vi "MC.SetWavelength.vi"(8 "error in (no error)":errorcluster, 10 "Wavelength, nm":T1, 11 "Measurement.Free":refnum<class "Measurement.Free.lvclass">) -> (0 "error out":errorcluster, 3 "Measurement.Free out":refnum<class "Measurement.Free.lvclass">)   [LabVIEW 2017, in "Measurement.Free.lvclass"]
doc: "---------------------------------------------------------------\nJKI State Machine Objects™\nhttp://jki.net/state-machine-objects/\nCopyright (C) 2005-2015, JKI <info@jki.net>\nALL RIGHTS RESERVEDJKI State Machine Objects (SMO) 1.0.0.4\nJKI - JKI\nCopyright (c) 2015, JKI"
uses:
  Measurement.Free.lvclass
  Typedefs/PrivateEvents--Measurement.Free.MC.SetWavelength.ctl
  Measurement.Free.lvclass/Measurement.Free.ctl
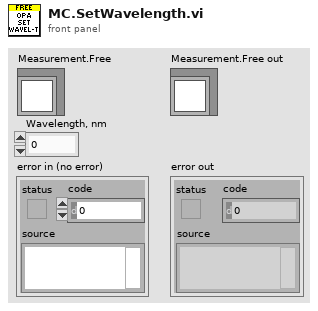
[diagram p1: front panel]
types:
  T1 = typedef "Measurement.Free.lvclass/PrivateEvents--Measurement.Free.MC.SetWavelength.ctl" = dbl
  T2 = typedef "Measurement.Free.lvclass/PrivateData--Ref.ctl" = refnum<data-value>
  T3 = typedef "Measurement.Free.lvclass/PrivateData--Cluster.ctl" = cluster{"Configuration":T4, "Dependencies":T17, "Private Events":T18}
  T4 = typedef "Measurement.Free.lvclass/Configuration--Cluster.ctl" = cluster{"Measurement.Type":T5, "Hardware":T6}
  T5 = typedef "Measurement.lvclass/Measurement.Type--Enum.ctl" = enum16{"Free", "I/V Curve", "Wavelength sweeping", "Photocurrent mapping"}
  T6 = typedef "Measurement.Free.lvclass/Configuration.Hardware--Cluster.ctl" = cluster{"SMU":T7, "LIA":T9, "OPM":T11, "OPA":T13, "MC":T15}
  T7 = typedef "Measurement.lvclass/Configuration.SMU--Cluster.ctl" = cluster{"Enable":bool, "SMU Model":string, "Configuration":T8}
  T8 = typedef "SMU.lvclass/Configuration--Cluster.ctl" = cluster{"VISA Resource":string, "Channel":string}
  T9 = typedef "Measurement.lvclass/Configuration.LIA--Cluster.ctl" = cluster{"Enable":bool, "LIA Model":string, "Configuration":T10}
  T10 = typedef "LIA.lvclass/Configuration--Cluster.ctl" = cluster{"VISA Resource":string}
  T11 = typedef "Measurement.lvclass/Configuration.OPM--Cluster.ctl" = cluster{"Enable":bool, "OPM Model":string, "Configuration":T12}
  T12 = typedef "OPM.lvclass/Configuration--Cluster.ctl" = cluster{"VISA Resource":string}
  T13 = typedef "Measurement.lvclass/Configuration.OPA--Cluster.ctl" = cluster{"Enable":bool, "OPA Model":string, "Configuration":T14}
  T14 = typedef "OPA.lvclass/Configuration--Cluster.ctl" = cluster{"Serial Number":string}
  T15 = typedef "Measurement.lvclass/Configuration.MC--Cluster.ctl" = cluster{"Enable":bool, "MC Model":string, "Configuration":T16}
  T16 = typedef "MC.lvclass/Configuration--Cluster.ctl" = cluster{"VISA Resource":string}
  T17 = typedef "Measurement.Free.lvclass/Dependencies--Cluster.ctl" = cluster{"SMU":refnum<class "SMU.lvclass">, "LIA":refnum<class "LIA.lvclass">, "OPM":refnum<class "OPM.lvclass">, "OPA":refnum<class "OPA.lvclass">, "MC":refnum<class "MC.lvclass">}
  T18 = typedef "Measurement.Free.lvclass/PrivateEvents--Cluster.ctl" = cluster{"SMU.SetVoltage":refnum<user-event>, "OPA.SetWavelength":refnum<user-event>, "OPA.SetShutterState":refnum<user-event>, "MC.SetWavelength":refnum<user-event>}
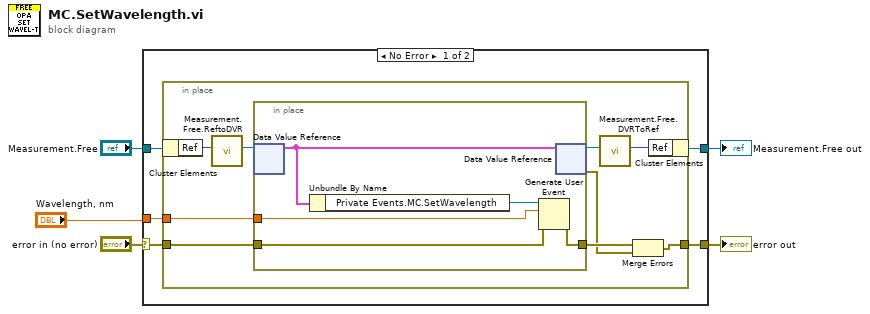
[diagram p0: block diagram]
diagram:
  n1 = case shown="No Error" "error in (no error)" {
    selector: "error in (no error)" -> [w8 w26]
    tunnel: [w7 w26] -> w4
    tunnel: [w9 w25] -> w5
    tunnel: "Measurement.Free" -> [w10 w25]
    tunnel: "Wavelength, nm" -> [w6 _]
    frame No Error {
      n2 = in-place {
        in-place-border: w8 -> [w19]
        in-place-border: [w16] -> w7
        in-place-border: w6 -> [w13]
        n3 = in-place-cluster #1(w10) -> ("Ref"=w15:u32)
        n4 = call "Measurement.Free.ReftoDVR.vi"("Ref"=w15) -> ("Ref"=w12:T2)  [unwired: 10 in]
        n5 = in-place {
          in-place-border: w19 -> [w22]
          in-place-border: [w21] -> w18
          in-place-border: w13 -> [w20]
          n6 = in-place-dvr #2(w12) -> (w24:T3)  [unwired: 1 out]
          n7 = Unbundle By Name(w24) -> ("Private Events.MC.SetWavelength"=w23:refnum<user-event>)
          n8 = Generate User Event(user event=w23, event data cluster=w20, error in=w22) -> (error out=w21:errorcluster)  [unwired: 1 in, 1 out]
          n9 = in-place-dvr #2(w24) -> (w14:T2, w17:errorcluster)
        }
        n10 = call "Measurement.Free.DVRToRef.vi"("Ref"=w14) -> ("Ref"=w11:u32)  [unwired: 10 in]
        n11 = Merge Errors(w18, w17) -> (w16:errorcluster)
        n12 = in-place-cluster #1("Ref"=w11) -> (w9:refnum<class "Measurement.Free.lvclass">)
      }
    }
    frame Error {
    }
  }
  "error out" <- w4
  "Measurement.Free out" <- w5
